vi "SetUpRings.vi"(0 "Center Hole":dbl=1.0 format="%.5f", 1 "Array":bool[](array[boolean]), 2 "Calc":u16(ring) items=["One way", "RT Single Rings", "R/T Full Aperture"], 5 "Variables":T2={"Number of rings"=1, "sound spd (cm/s)"=150000, "z span (cm)"=4.0, "z steps"=20, "y spacing (cm)"=0.01, "y steps"=50, "time step (s)"=1e-08, "z"=0.0, "y"=0.0, "ref delay"=0.0, "freq (MHz)"=4.71, "cycles"=300.0} {"freq (MHz)" format="%.2f"; "z span (cm)" format="%.2f"; "y" format="%.2f"; "ref delay" format="%.2f"; "y spacing (cm)" format="%.2f"; "z" format="%.2f"; "time step (s)" format="%.2e"}, 7 "Gain":dbl[](array[numeric]) format="%.2f", 9 "Trans Geometry":T4={"Radius"=4.8, "a"=1.0, "focus location"=12.0} {"focus location" format="%.2f"; "a" format="%.4f"; "Radius" format="%.2f"}, 11 "kerf space (cm)":dbl format="%.5f", 12 "Kerf?":bool, 13 "Drive waveform":sgl[](array[numeric])=[1.562, 3.125, 3.125, 3.906, 3.125, 1.562, 1.562, 2.344, 3.125, 3.125, 3.125, 3.906, 4.687, 4.687, 5.469, 4.687, 3.125, 1.562, 1.562, 0.781, 1.562, 1.562, 1.562, 3.125, 3.125, 2.344, 1.562, 3.125, 2.344, 0.781, 0.0, 0.0, -0.781, -0.781, 0.0, 1.562, 3.125, 3.125, 3.125, 3.125, 2.344, 1.562, -0.781, -0.781, 0.781, 3.125, 3.125, 3.906, 3.906, 3.906, 4.687, 3.125, 1.562, 1.562, 2.344, 2.344, 2.344, 3.125, 3.906, 3.125, 2.344, 0.781, 0.0, -0.781, 0.781, 0.781, 0.781, 0.781, 0.781, 0.0, 0.0, 0.0, 0.0, 0.0, -0.781, -1.562, -3.125, -3.125, -4.687, -3.906, -7.031, -10.156, -12.5, -16.406, -18.75, -22.656, -24.219, -18.75, -9.375, 7.812, 28.125, 47.656, 65.625, 73.437, 73.437, 66.406, 53.906, 41.406, 27.344, 14.844, 3.906, -5.469, -14.062, -22.656, -25.781, -26.562, -25.0, -24.219, -21.875, -21.875, -25.0, -28.125, -32.812, -37.5, -44.531, -46.875, -43.75, -32.031, -15.625, 3.125, 25.0, 39.062, 47.656, 50.0, 45.312, 35.156, 24.219, 13.281, 4.687, -3.906, -9.375, -12.5, -13.281, -17.187, -17.187, -14.062, -7.812, -3.125, 1.562, 0.781, -0.781, -3.906, -6.25, -8.594, -8.594, -9.375, -7.031, -3.125, 0.0, 4.687, 6.25, 8.594, 8.594, 10.937, 10.156, 10.156, 9.375, 7.812, 4.687, 1.562, -0.781, -2.344, -3.125, -3.906, -3.125, -2.344, -0.781, 1.562, 3.125, 3.125, 1.562, 1.562, 1.562, 1.562, 1.562, 2.344, 3.906, 3.125, 3.125, 3.125, 2.344, 2.344, 0.781, -0.781, 0.0, 3.125, 4.687, 6.25, 5.469, 5.469, 6.25, 6.25, 6.25, 4.687, 6.25, 7.031, 6.25, 6.25, 6.25, 9.375, 9.375, 7.812, 7.031, 7.031, 7.031, 5.469, 5.469, 5.469, 5.469, 5.469, 4.687, 3.125, 3.125, 2.344, 2.344, 1.562, 3.125, 5.469, 5.469, 5.469, 5.469, 5.469, 5.469, 4.687, 3.906, 3.906, 3.125, 3.125, 3.906, 2.344, 1.562, 2.344, 2.344, 3.125, 3.125, 3.125, 3.125, 3.125, 1.562, 0.781, 0.0, 0.781, 0.0] format="%.2f") -> (3 "annuli list":string[](array[string]), 4 "Rings":T3(array[cluster]) {"focus delay abs (s)" format="%.2e"; "Waveform" format="%.2f"; "Annular rings"."a" format="%.2f"; "Annular rings"."Radius" format="%.2f"}, 6 "projected ring locations":string, 8 "rings (m)":dbl[](array[numeric]), 10 "Variables out":T2={"Number of rings"=1, "sound spd (cm/s)"=150000, "z span (cm)"=4.0, "z steps"=20, "y spacing (cm)"=0.01, "y steps"=50, "time step (s)"=1e-08, "z"=0.0, "y"=0.0, "ref delay"=0.0, "freq (MHz)"=4.71, "cycles"=300.0} {"freq (MHz)" format="%.2f"; "z span (cm)" format="%.2f"; "y" format="%.2f"; "ref delay" format="%.2f"; "y spacing (cm)" format="%.2f"; "z" format="%.2f"; "time step (s)" format="%.2e"}, 15 "Rings":picture)   [LabVIEW 2022 SP3]
uses:
  <vilib>/Analysis/NI_AALPro.lvlib
panel:
  out "Spectrum":T1(graph)
  out "delays rel":dbl[](array[numeric]) format="%.2e"
  out "flattened locations":string
  out "Waveform Graph":sgl[][](graph)
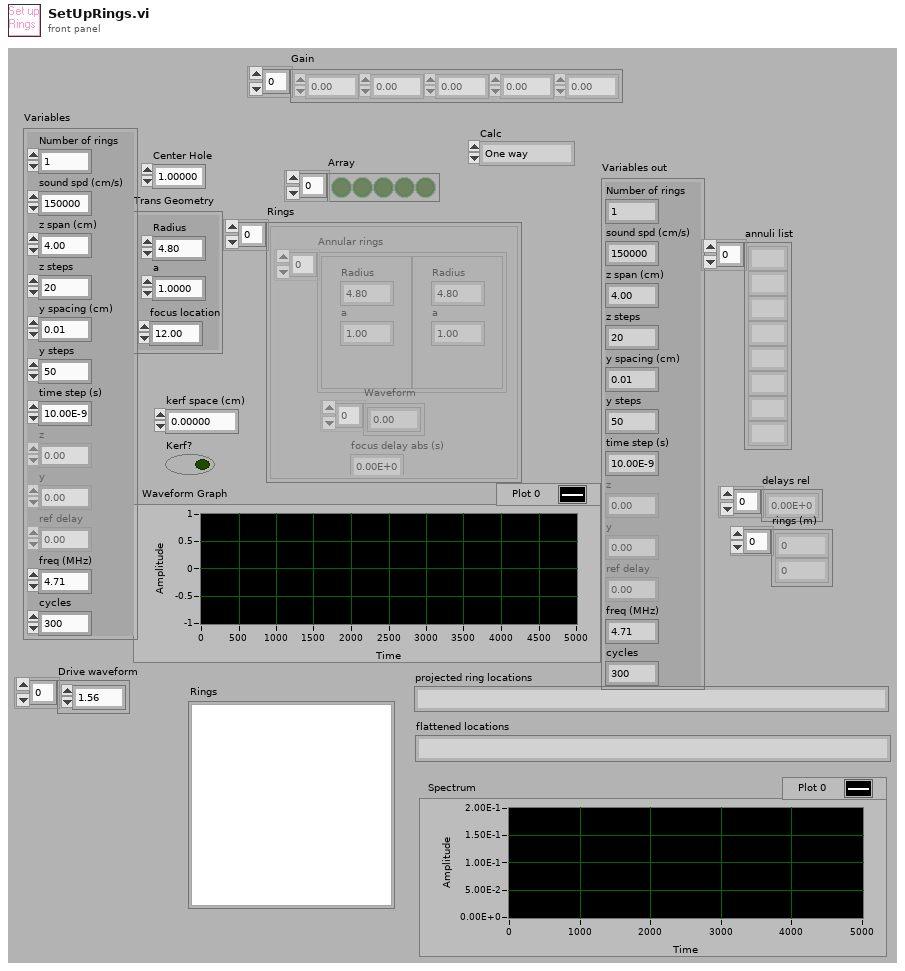
[diagram p1: front panel]
types:
  T1 = cluster{i32, "df":dbl, "Power Spectrum (V^2 rms)":dbl[]}
  T2 = cluster{"Number of rings":i32, "sound spd (cm/s)":i32, "z span (cm)":dbl, "z steps":i32, "y spacing (cm)":dbl, "y steps":i32, "time step (s)":sgl, "z":dbl, "y":dbl, "ref delay":dbl, "freq (MHz)":dbl, "cycles":sgl}
  T3 = cluster{"Annular rings":cluster{"Radius":dbl, "a":dbl}[], "Waveform":dbl[], "focus delay abs (s)":dbl}[]
  T4 = cluster{"Radius":dbl, "a":dbl, "focus location":dbl}
  T5 = cluster{"appended array":cluster{"R":dbl, "a":dbl}[], sgl[], dbl}
  T6 = cluster{"appended array":cluster{"R":dbl, "a":dbl}[], sgl[], dbl}[]
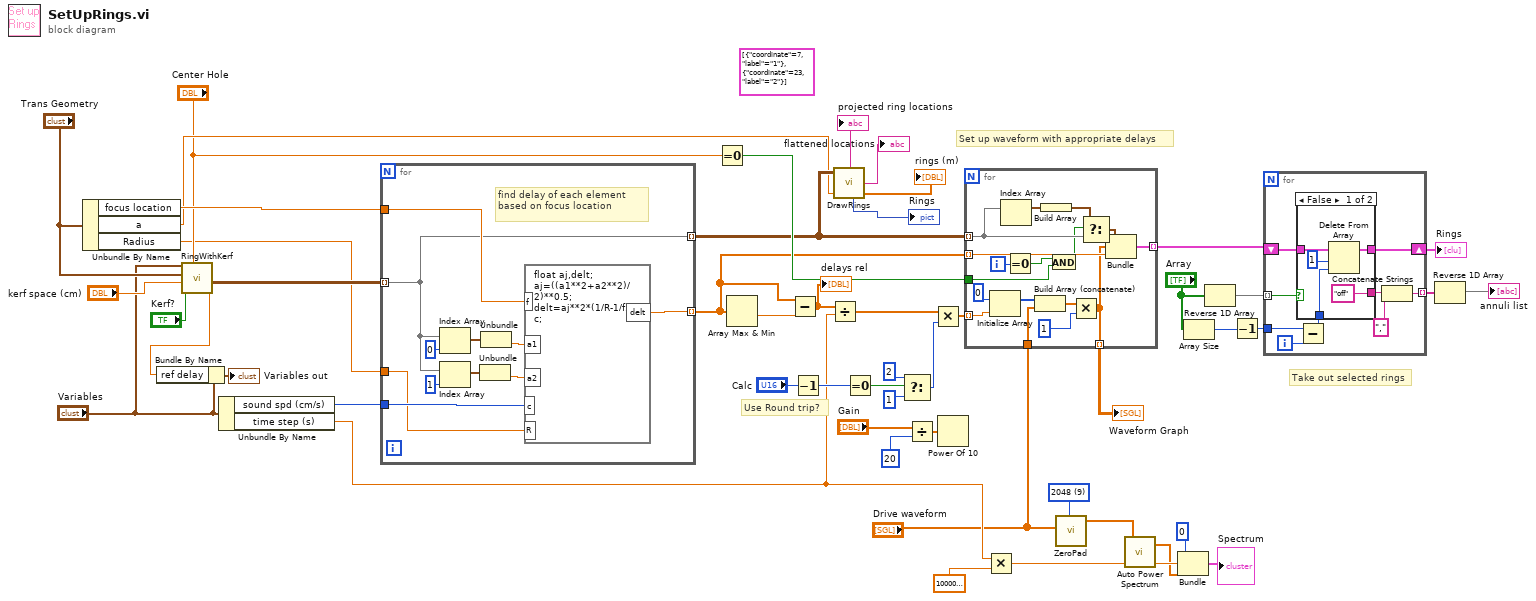
[diagram p0: block diagram]
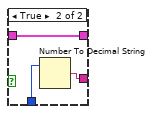
[diagram p2: hidden frame]
diagram:
  w5 = u16 9 items=["next 2^n", "8", "16", "32", "64", "128", "256", "512", "1024", "2048"] ("FFT size")
  (unwired) cluster{"coordinate":i16, "label":string}[] [{"coordinate"=7, "label"="1"}, {"coordinate"=23, "label"="2"}] ("scale specs")
  # "Use Round trip?"
  # "Take out selected rings"
  # "Set up waveform with appropriate delays"
  n1 = Unbundle By Name("Trans Geometry") -> ("focus location"=w49:dbl, "a"=w44:dbl, "Radius"=w7:dbl)
  n2 = call "RingWithKerf.vi"("Center Hole"="Center Hole", "kerf?"="Kerf?", "kerf space (cm)"="kerf space (cm)", "Trans Geometry"="Trans Geometry", "Variables"="Variables") -> ("refdelay"=w11:dbl, "appended array"=w34:cluster{"R":dbl, "a":dbl}[][])  [unwired: 2 in, 1 out]
  n3 = Bundle By Name(cluster="Variables", "ref delay"=w11) -> (→"Variables out":T2)
  n4 = Unbundle By Name("Variables") -> ("sound spd (cm/s)"=w51:i32, "time step (s)"=w6:sgl)
  n5 = for {
    tunnel: w51 -> [w56]
    tunnel: [w55] -> w28 mode=indexing
    tunnel: [w53] -> w46 mode=indexing
    tunnel: w49 -> [w54]
    tunnel: w34 -> [w53] mode=indexing
    tunnel: w7 -> [w52]
    # "find delay of each element based on focus location"
    n6 = Index Array(array=w53, index=0) -> (element=w60:cluster{"R":dbl, "a":dbl})
    n7 = Index Array(array=w53, index=1) -> (element=w59:cluster{"R":dbl, "a":dbl})
    n8 = Unbundle(w59) -> ("a"=w57:dbl)  [unwired: 1 out]
    n9 = Unbundle(w60) -> ("a"=w58:dbl)  [unwired: 1 out]
    n10 = formula code="float aj,delt;\naj=((a1**2+a2**2)/2)**0.5;\ndelt=aj**2*(1/R-1/f)/2/c;"("R"=w52, "f"=w54, "a1"=w58, "a2"=w57, "c"=w56) -> ("delt"=w55:dbl)
  }
  n11 = Equal To 0?(x="Center Hole") -> (x = 0?=w47:bool)
  n12 = Array Max & Min(array=w28) -> (min value=w50:dbl)  [unwired: 3 out]
  n13 = Subtract(x=w28, y=w50) -> (x-y=w29:dbl[])
  "delays rel" <- w29
  n14 = Decrement(x="Calc") -> (x-1=w19:u16)
  n15 = Divide(x=w29, y=w6) -> (x/y=w30:dbl[])
  n16 = call "DrawRings.vi"("Ring Array"=w46, "a"=w44) -> ("ring locations (a)"=→"projected ring locations":string, "flattened locations"=→"flattened locations":string, "Ring Pict"=→"Rings":picture, "rings (m)"=→"rings (m)":dbl[])  [unwired: 4 out]
  n17 = Equal To 0?(x=w19) -> (x = 0?=w18:bool)
  n18 = Select(t=2, s=w18, f=1) -> (s? t:f=w21:i32)
  n19 = Divide(x="Gain", y=20) -> (x/y=w25:dbl[])
  n20 = Multiply(x=w30, y=w21) -> (x*y=w24:dbl[])
  n21 = Power Of 10(x=w25) -> ()  [unwired: 1 out]
  n22 = for {
    tunnel: w46 -> [w71] mode=indexing
    tunnel: w28 -> [w79] mode=indexing
    tunnel: "Drive waveform" -> [w74]
    tunnel: [w77] -> w43 mode=indexing
    tunnel: w24 -> [w76] mode=indexing
    tunnel: w47 -> [w67]
    tunnel: [w64] -> w3 mode=indexing
    i -> [w72]
    n23 = Initialize Array(0, w76) -> (w75:i32[])
    n24 = Index Array(array=w71) -> (element=w70:cluster{"R":dbl, "a":dbl})  [unwired: 1 in]
    n25 = Equal To 0?(x=w72) -> (x = 0?=w68:bool)
    n26 = Build Array (concatenate)(w75, w74) -> (w65:sgl[])
    n27 = Build Array(w70) -> (w69:cluster{"R":dbl, "a":dbl}[])
    n28 = And(x=w68, y=w67) -> (x .and. y?=w66:bool)
    n29 = Multiply(x=w65, y=1) -> (x*y=w64:sgl[])
    n30 = Select(t=w69, s=w66, f=w71) -> (s? t:f=w73:cluster{"R":dbl, "a":dbl}[])
    n31 = Bundle("appended array"=w73, w64, w79) -> (w77:T5)  [unwired: 1 out]
  }
  "Waveform Graph" <- w3
  n32 = Multiply(x=w6, y=1000000.0) -> (x*y=w17:dbl)
  n33 = call "ZeroPad.vi"("Input Array"="Drive waveform", "FFT size"=w5) -> ("Ouput Array"=w4:dbl[])  [unwired: 4 out]
  n34 = call <vilib>:"Auto Power Spectrum.vi"("dt"=w17, "Signal (V)"=w4) -> ("df"=w16:dbl, "Power Spectrum (V^2 rms)"=w15:dbl[])
  n35 = Bundle(0, "df"=w16, "Power Spectrum (V^2 rms)"=w15) -> (→"Spectrum":T1)  [unwired: 1 out]
  n36 = Array Size(array="Array") -> (size(s)=w38:i32)
  n37 = Reverse 1D Array(array="Array") -> (reversed array=w41:bool[])
  n38 = Decrement(x=w38) -> (x-1=w36:i32)
  n39 = for {
    shift-right: [w87] -> w42
    shift-left: w43 -> [w88]
    tunnel: w41 -> [w86] mode=indexing
    tunnel: [w84] -> w40 mode=indexing
    tunnel: w36 -> [w81]
    i -> [w82]
    n40 = Subtract(x=w81, y=w82) -> (x-y=w80:i32)
    n41 = case shown="False" w86 {
      tunnel: [w93 w96] -> w87
      tunnel: w80 -> [w90 w95]
      tunnel: w88 -> [w91 w96]
      tunnel: ["off" w94] -> w85
      frame False {
        n42 = Delete From Array(array=w91, length=1, index=w90) -> (array with subset deleted=w93:T6)  [unwired: 1 out]
      }
      frame True {
        n43 = Number To Decimal String(number=w95) -> (decimal integer string=w94:string)  [unwired: 1 out]
      }
    }
    n44 = Concatenate Strings(w85, ",") -> (w84:string)
  }
  "Rings" <- w42
  n45 = Reverse 1D Array(array=w40) -> (reversed array=→"annuli list":string[])
